vi "Read_Selected_channels.vi"(0 "Filename":path, 1 "Valid Channel Options":string[][](array[string]), 2 "Template Names":string[](array[string]), 3 "Data string":string, 5 "All Channels Present":string[](array[string]), 6 "End Of File already Reached?":bool, 9 "Start of data (bytes)":i32, 11 "Column OK in":bool[](array[boolean]), 12 "Filetype":string, 14 "Ignore When":string[][](array[string])) -> (4 "Non-Blank Rows":i32[](array[numeric]), 10 "Output Values":string[][](array[string]), 15 "Column OK Out":bool[](array[boolean]))   [LabVIEW 2010]
uses:
  Data_plotting_vis/Results_plotter_Global.vi
panel:
  out "Case":string
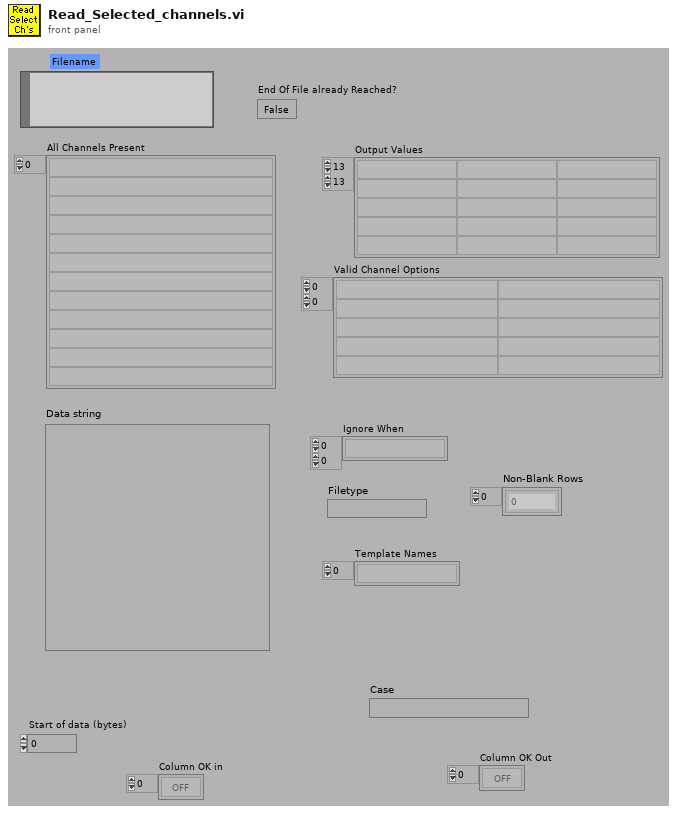
[diagram p1: front panel]
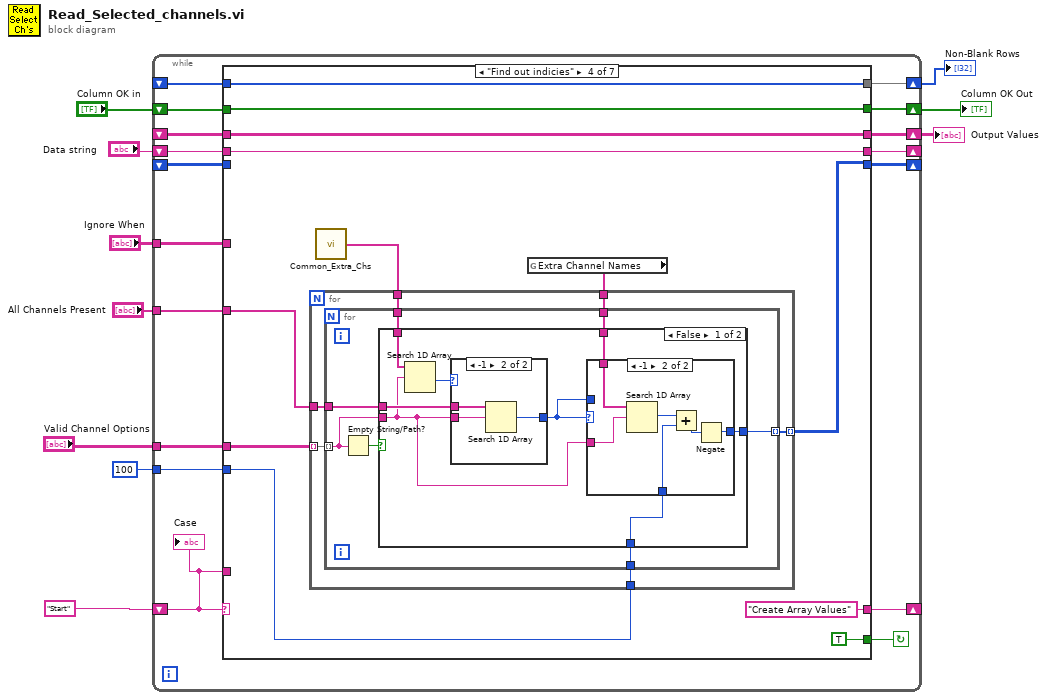
[diagram p0: block diagram]
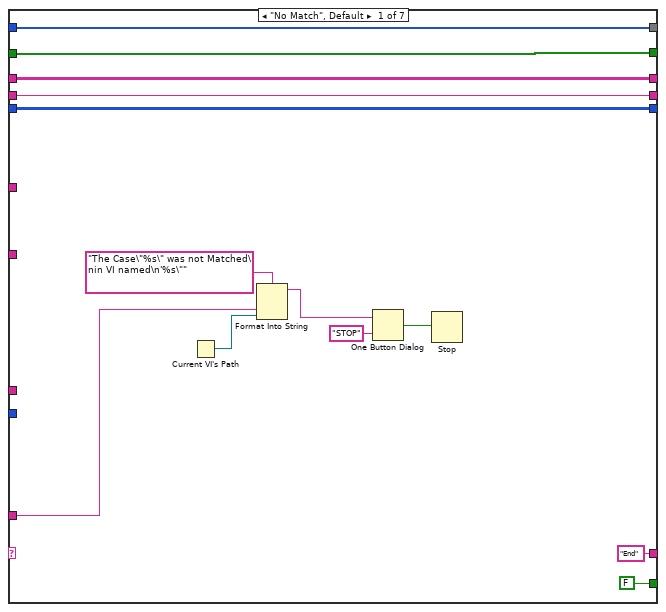
[diagram p2: hidden frame]
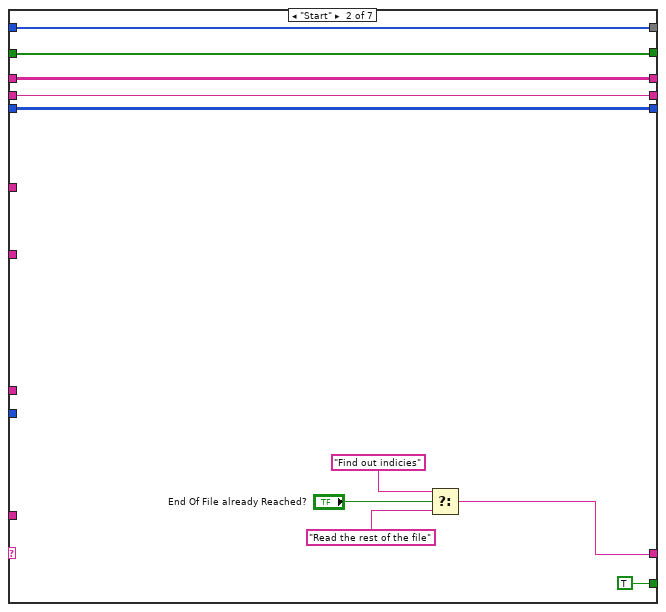
[diagram p3: hidden frame]
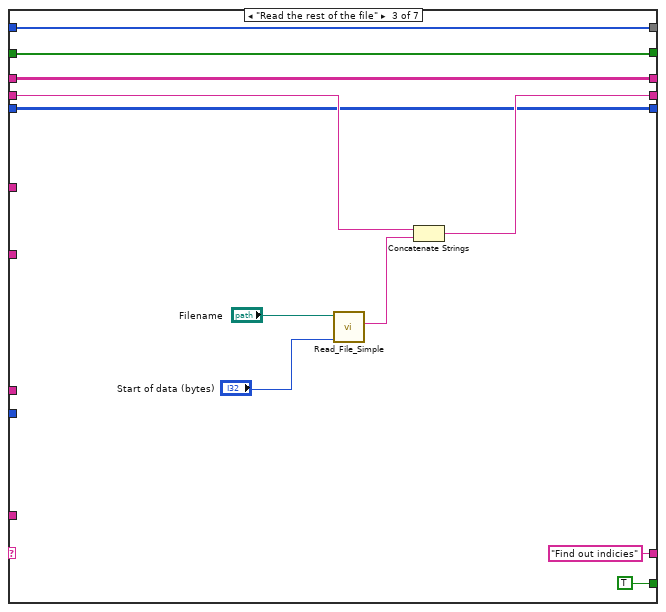
[diagram p4: hidden frame]
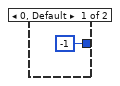
[diagram p5: hidden frame]
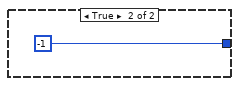
[diagram p7: hidden frame]
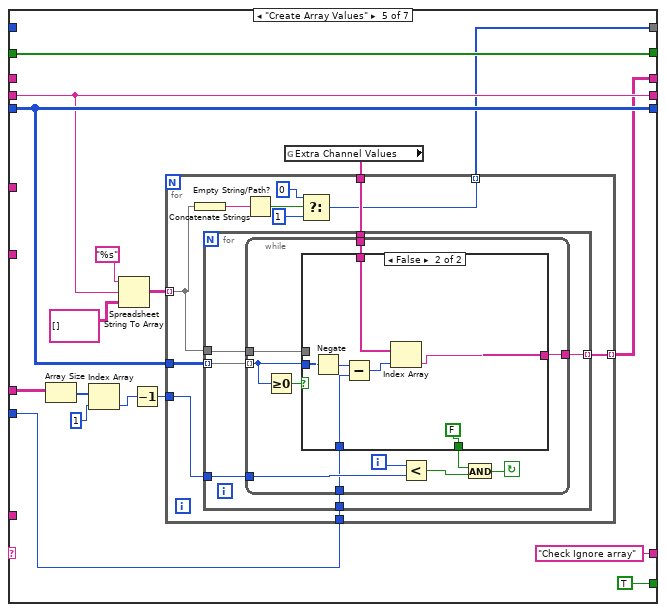
[diagram p8: hidden frame]
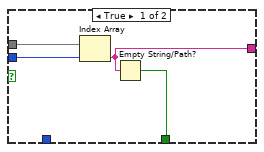
[diagram p9: hidden frame]
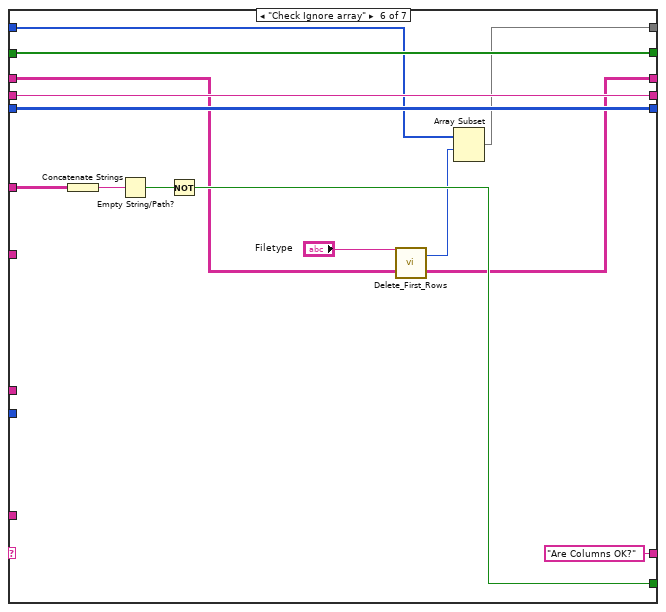
[diagram p10: hidden frame]
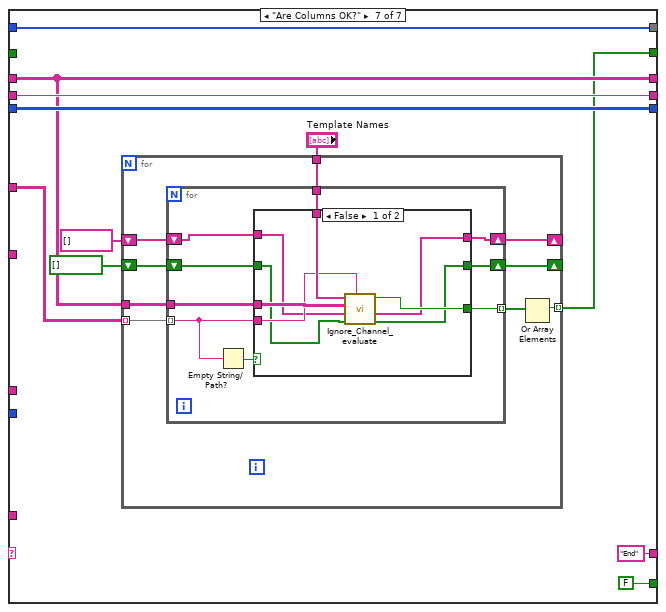
[diagram p11: hidden frame]
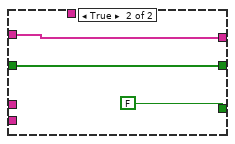
[diagram p12: hidden frame]
diagram:
  n1 = while {
    shift-left: "Column OK in" -> [w13]
    shift-right: [w14] -> w3
    tunnel: "Ignore When" -> [w15]
    shift-left: _ -> [w16]
    shift-right: [w17] -> w5
    tunnel: 100 ("y") -> [w18]
    tunnel: "Valid Channel Options" -> [w19]
    tunnel: "All Channels Present" -> [w20]
    shift-left: "Data string" -> [w22]
    shift-right: [w21] -> _
    shift-left: _ -> [w24]
    shift-right: [w23] -> _
    shift-left: "Start" -> [w26]
    shift-right: [w25] -> _
    shift-right: [w12] -> w1
    shift-left: _ -> [w11]
    stop <- w27 continue-if-true
    n2 = case shown="\"Find out indicies\"" w26 {
      tunnel: [FALSE ("Results File?") TRUE ("Results File?") TRUE ("Results File?") TRUE ("Results File?") TRUE ("Results File?") w170 FALSE ("Results File?")] -> w27
      tunnel: w26 -> [w35 _ _ _ _ _ _]
      tunnel: ["End" w45 "Find out indicies" ("f") "Create Array Values" ("f") "Check Ignore array" ("f") "Are Columns OK?" "End"] -> w25
      tunnel: w24 -> [w32 w44 w55 _ w114 w175 w186]
      tunnel: [w32 w44 w55 w67 w114 w175 w186] -> w23
      tunnel: w22 -> [w31 w49 w56 w73 w110 w174 w185]
      tunnel: [w31 w49 w57 w73 w110 w174 w185] -> w21
      tunnel: w20 -> [_ _ _ w68 _ _ _]
      tunnel: w19 -> [_ _ _ w70 w116 _ _]
      tunnel: w18 -> [_ _ _ w66 w120 _ _]
      tunnel: [w30 w43 w53 w65 w109 w167 w183] -> w17
      tunnel: w16 -> [w30 w43 w53 w65 _ w166 w183]
      tunnel: w15 -> [_ _ _ _ _ w173 w182]
      tunnel: [w29 w42 w52 w64 w108 w169 w180] -> w14
      tunnel: w13 -> [w29 w42 w52 w64 w108 w169 _]
      tunnel: [w28 w41 w51 w63 w107 w163 w177] -> w12
      tunnel: w11 -> [w28 w41 w51 w63 _ w164 w177]
      frame "No Match", Default {
        n3 = Current VI's Path() -> (path=w36:path)
        n4 = Format Into String(format string="The Case\"%s\" was not Matched\nin VI named\n'%s\"" ("Format String"), w35, w36) -> (resulting string=w39:string)  [unwired: 2 in, 1 out]
        n5 = One Button Dialog(message=w39, button name ("OK")="STOP") -> (true=w37:bool)
        n6 = Stop(stop? (T)=w37) -> ()
      }
      frame "Start" {
        n7 = Select(t="Find out indicies" ("f"), s="End Of File already Reached?", f="Read the rest of the file") -> (s? t:f=w45:string)
      }
      frame "Read the rest of the file" {
        n8 = call "Read_File_Simple.vi"("Filename"="Filename", "pos offset (bytes:0)"="Start of data (bytes)") -> ("string"=w58:string)  [unwired: 1 in, 7 out]
        n9 = Concatenate Strings(w56, w58) -> (w57:string)
      }
      frame "Find out indicies" {
        n10 = call "Common_Extra_Chs.vi"() -> ("Common Extra Channels"=w62:string[])
        n11 = global read "Results_plotter_Global.vi" "Extra Channel Names"() -> (w69:string[])
        n12 = for {
          tunnel: w68 -> [w79]
          tunnel: w70 -> [w78] mode=indexing
          tunnel: [w77] -> w67 mode=indexing
          tunnel: w66 -> [w76]
          tunnel: w69 -> [w75]
          tunnel: w62 -> [w74]
          n13 = for {
            tunnel: w78 -> [w84] mode=indexing
            tunnel: w79 -> [w86]
            tunnel: [w85] -> w77 mode=indexing
            tunnel: w76 -> [w82]
            tunnel: w75 -> [w81]
            tunnel: w74 -> [w80]
            n14 = Empty String/Path?(string/path=w84) -> (empty?=w83:bool)
            n15 = case shown="False" w83 {
              tunnel: w86 -> [w94 _]
              tunnel: [w93 -1 ("index of element")] -> w85
              tunnel: w84 -> [w88 _]
              tunnel: w82 -> [w91 _]
              tunnel: w81 -> [w90 _]
              tunnel: w80 -> [w89 _]
              frame False {
                n16 = Search 1D Array(1D array=w89, element=w88) -> (index of element=w87:i32)  [unwired: 1 out]
                n17 = case shown="-1" w87 {
                  tunnel: w94 -> [_ w98]
                  tunnel: [-1 ("index of element") w97] -> w92
                  tunnel: w88 -> [_ w96]
                  frame 0, Default {
                  }
                  frame -1 {
                    n18 = Search 1D Array(1D array=w98, element=w96) -> (index of element=w97:i32)  [unwired: 1 out]
                  }
                }
                n19 = case shown="-1" w92 {
                  tunnel: w88 -> [_ w105]
                  tunnel: [w99 w102] -> w93
                  tunnel: w92 -> [w99 _]
                  tunnel: w91 -> [_ w101]
                  tunnel: w90 -> [_ w100]
                  frame 0, Default {
                  }
                  frame -1 {
                    n20 = Search 1D Array(1D array=w100, element=w105) -> (index of element=w104:i32)  [unwired: 1 out]
                    n21 = Add(x=w104, y=w101) -> (x+y=w103:i32)
                    n22 = Negate(x=w103) -> (-x=w102:i32)
                  }
                }
              }
              frame True {
              }
            }
          }
        }
      }
      frame "Create Array Values" {
        n23 = Array Size(array=w116) -> (size(s)=w119:i32[])
        n24 = Index Array(array=w119, index=1 ("Index")) -> (element=w117:i32)
        n25 = Spreadsheet String To Array(format string="%s", spreadsheet string=w110, array type (2D Dbl)=string[][] []) -> (array=w111:string[][])  [unwired: 1 out]
        n26 = Decrement(x=w117) -> (x-1=w115:i32)
        n27 = global read "Results_plotter_Global.vi" "Extra Channel Values"() -> (w121:string[])
        n28 = for {
          tunnel: w114 -> [w134]
          tunnel: w111 -> [w128] mode=indexing
          tunnel: [w133] -> w109 mode=indexing
          tunnel: w120 -> [w132]
          tunnel: w121 -> [w131]
          tunnel: w115 -> [w130]
          tunnel: [w126] -> w107 mode=indexing
          n29 = Concatenate Strings(w128) -> (w129:string)
          n30 = for {
            tunnel: w134 -> [w138] mode=indexing
            tunnel: w128 -> [w140]
            tunnel: [w139] -> w133 mode=indexing
            tunnel: w130 -> [w137]
            tunnel: w132 -> [w136]
            tunnel: w131 -> [w135]
            n31 = while {
              tunnel: w135 -> [w141]
              tunnel: w136 -> [w142]
              tunnel: w137 -> [w148]
              tunnel: w138 -> [w144] mode=indexing
              tunnel: [w150] -> w139
              tunnel: w140 -> [w151]
              i -> [w149]
              stop <- w146 continue-if-true
              n32 = Greater Or Equal To 0?(x=w144) -> (x >= 0?=w143:bool)
              n33 = case shown="False" w143 {
                tunnel: w151 -> [w155 _]
                tunnel: [w153 w162] -> w150
                tunnel: w144 -> [w154 w161]
                tunnel: [w152 FALSE] -> w145
                tunnel: w142 -> [_ w159]
                tunnel: w141 -> [_ w156]
                frame True {
                  n34 = Index Array(array=w155, index=w154) -> (element=w153:string)
                  n35 = Empty String/Path?(string/path=w153) -> (empty?=w152:bool)
                }
                frame False {
                  n36 = Negate(x=w161) -> (-x=w160:i32)
                  n37 = Subtract(x=w160, y=w159) -> (x-y=w158:i32)
                  n38 = Index Array(array=w156, index=w158) -> (element=w162:string)
                }
              }
              n39 = Less?(x=w149, y=w148) -> (x < y?=w147:bool)
              n40 = And(x=w145, y=w147) -> (x .and. y?=w146:bool)
            }
          }
          n41 = Empty String/Path?(string/path=w129) -> (empty?=w127:bool)
          n42 = Select(t=0, s=w127, f=1) -> (s? t:f=w126:i32)
        }
      }
      frame "Check Ignore array" {
        n43 = Concatenate Strings(w173) -> (w172:string)
        n44 = Empty String/Path?(string/path=w172) -> (empty?=w171:bool)
        n45 = Not(x=w171) -> (.not. x?=w170:bool)
        n46 = call "Delete_First_Rows.vi"("Data In"=w166, "File Type"="Filetype") -> ("Data Out"=w167:string[][], "Rows removed"=w165:i32)
        n47 = Array Subset(array=w164, index=w165) -> (w163:i32[])  [unwired: 1 in]
      }
      frame "Are Columns OK?" {
        n48 = for {
          tunnel: "Template Names" -> [w196]
          tunnel: w183 -> [w195]
          tunnel: w182 -> [w194] mode=indexing
          tunnel: [w192] -> w180 mode=indexing
          shift-right: [w191] -> _
          shift-left: string[] [] ("Commands Out") -> [w189]
          shift-right: [w190] -> _
          shift-left: bool[] [] ("Ignore array out") -> [w188]
          n49 = for {
            tunnel: w196 -> [w205]
            tunnel: w195 -> [w204]
            tunnel: [w202] -> w193 mode=indexing
            tunnel: w194 -> [w201] mode=indexing
            shift-right: [w200] -> w191
            shift-left: w189 -> [w198]
            shift-right: [w199] -> w190
            shift-left: w188 -> [w197]
            n50 = Empty String/Path?(string/path=w201) -> (empty?=w203:bool)
            n51 = case shown="False" w203 {
              tunnel: w205 -> [w213 _]
              tunnel: w204 -> [w212 _]
              tunnel: w201 -> [w211 _]
              tunnel: [w210 FALSE ("Column OK")] -> w202
              tunnel: [w209 w215] -> w200
              tunnel: [w208 w214] -> w199
              tunnel: w198 -> [w207 w215]
              tunnel: w197 -> [w206 w214]
              frame False {
                n52 = call "Ignore_Channel_evaluate.vi"("Ignore When String"=w211, "Ignore array"=w206, "Commands in"=w207, "Data"=w212, "Template Names"=w213) -> ("Ignore array out"=w208:bool[], "Commands Out"=w209:string[], "Ignore Column"=w210:bool)  [unwired: 4 out]
              }
              frame True {
              }
            }
          }
          n53 = Or Array Elements(Boolean array=w193) -> (logical OR=w192:bool)
        }
      }
    }
    "Case" <- w26
  }
  "Output Values" <- w5
  "Column OK Out" <- w3
  "Non-Blank Rows" <- w1
